vi "SpecificTargetIP.vi"(8 "error in (no error)":errorcluster, 10 "Action":enum16{"Clear", "Get", "Set"}(ring), 11 "IP or Hostname in":string) -> (0 "error out":errorcluster, 3 "IP or Hostname out":string)   [LabVIEW 2021, in "myRIOMetaDataObj.lvclass"]
uses:
  myRIOMetaDataObj.lvclass
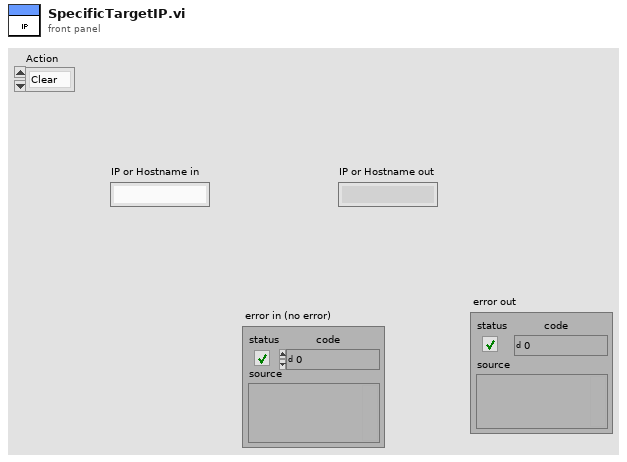
[diagram p1: front panel]
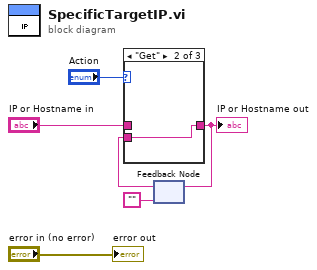
[diagram p0: block diagram]
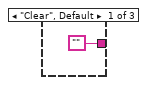
[diagram p2: hidden frame]
diagram:
  n1 = feedback #1("") -> (w3:string)
  n2 = case shown="\"Get\"" "Action" {
    tunnel: ["" w8 w9] -> w4
    tunnel: "IP or Hostname in" -> [_ _ w9]
    tunnel: w3 -> [_ w8 _]
    frame "Clear", Default {
    }
    frame "Get" {
    }
    frame "Set" {
    }
  }
  "IP or Hostname out" <- w4
  n3 = feedback-in #1(w4) -> ()
  "error out" <- "error in (no error)"
